vi "PicturetoIMAQImage.vi"() -> ()   [LabVIEW 2011]
uses:
  <vilib>/vision/Contour.llb/IMAQ Connect Range Setting.ctl
  <vilib>/vision/NI_Vision_Development_Module.lvlib
panel:
  in  "Curve Connection":T1[](array[typedef]) {"Max" format="%.2f"; "Min" format="%.2f"; "Match Constraints" items=["Distance (pixel)", "Angle Difference (degrees)", "Connectivity Distance (pixel)", "Gradient Difference (degrees)"]}
  out "Edge":T2(plugin-control)
  out "Input":T2(plugin-control)
  in  "Image Path":path=path "c:/kai.jpg"
  # "Range"
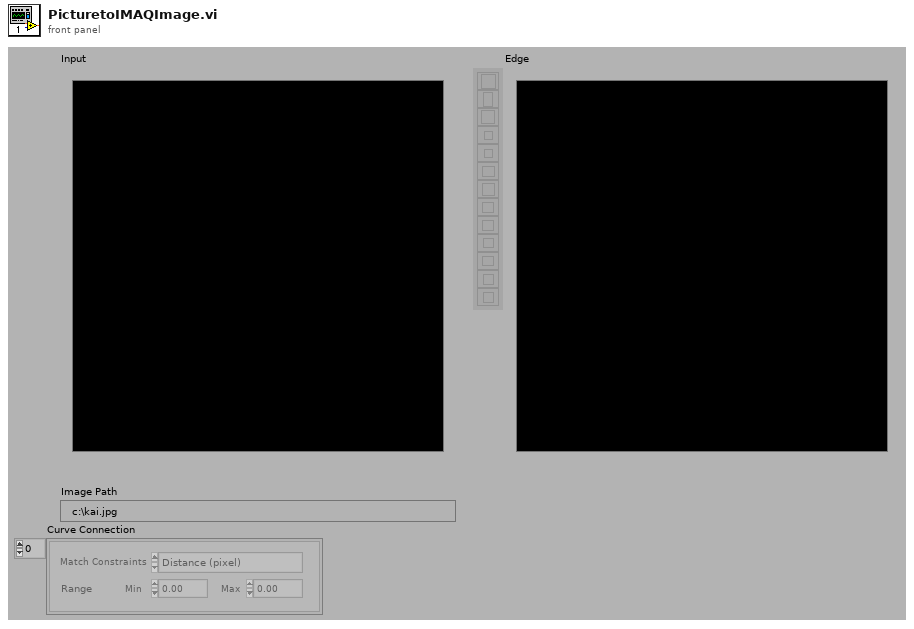
[diagram p1: front panel]
types:
  T1 = typedef "IMAQ Connect Range Setting.ctl" = cluster{"Match Constraints":u32, "Min":dbl, "Max":dbl}
  T2 = typedef "IMAQ Image.ctl" = refnum<image>
  T3 = enum16{"Rect Left To Right", "Rect Right To Left", "Rect Top To Bottom", "Rect Bottom To Top", "Annulus Inner To Outer", "Annulus Outer To Inner", "Annulus Start Angle To End Angle", "Annulus End Angle To Start Angle"}
  T4 = cluster{"Global Rectangle":i32[], "Contours":cluster{"Contour Type":u32, "ROI Type":u32, "Points":i32[]}[]}
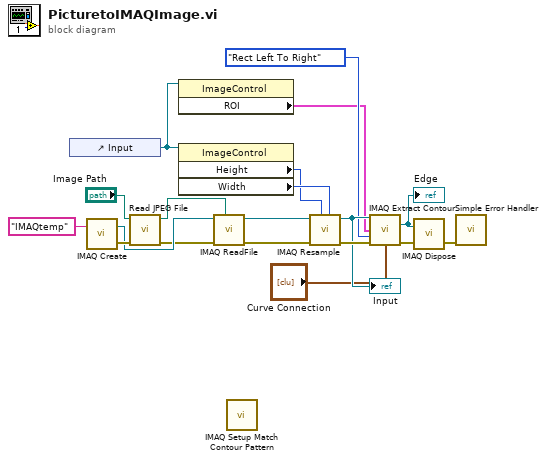
[diagram p0: block diagram]
diagram:
  n1 = control-ref of="Input"() -> (w3:refnum<vi>)
  n2 = call "IMAQ Create"("Image Name"="IMAQtemp") -> ("New Image"=w16:T2, "error out"=w18:errorcluster)  [unwired: 3 in, 1 out]
  n3 = call <vilib>:"Read JPEG File.vi"("error in (no error)"=w18, "path to JPEG file"="Image Path") -> ("error out"=w15:errorcluster, "path"=w14:path)  [unwired: 7 in, 1 out]
  n4 = property class="ImageControl"(reference=w3) -> ("ROI"=w2:T4)  [unwired: 1 in, 2 out]
  n5 = property class="ImageControl"(reference=w3) -> ("Height"=w9:u32, "Width"=w10:u32)  [unwired: 1 in, 2 out]
  n6 = call "IMAQ ReadFile"("File Path"=w14, "error in (no error)"=w15, "Image"=w16) -> ("error out"=w12:errorcluster, "Image Out"=w13:T2)  [unwired: 2 in, 5 out]
  n7 = call "IMAQ Setup Match Contour Pattern"() -> ()  [unwired: 10 in, 2 out]
  n8 = call "IMAQ Resample"("X Resolution"=w10, "Y Resolution"=w9, "error in (no error)"=w12, "Image Src"=w13) -> ("error out"=w6:errorcluster, "Image Dst Out"=w5:T2)  [unwired: 6 in]
  "Input" <- w5
  n9 = call "IMAQ Extract Contour"("Source Image"=w5, "ROI Descriptor"=w2, "Search Direction"=T3."Rect Left To Right", "error in (no error)"=w6, "Curve Connection"="Curve Connection") -> ("Contour Image Out"=w8:T2, "error out"=w7:errorcluster)  [unwired: 6 in, 3 out]
  "Edge" <- w8
  n10 = call "IMAQ Dispose"("Image"=w8, "error in (no error)"=w7) -> ("error out"=w11:errorcluster)  [unwired: 4 in]
  n11 = call <vilib>:"Simple Error Handler.vi"("error in (no error)"=w11) -> ()  [unwired: 4 in, 5 out]
